vi "RIGOL DM3058 Read Single.vi"() -> ()   [LabVIEW 2018]
doc: "This example shows how to configure a measurement and take a reading."
uses:
  <instrlib>/RIGOL DM3058/RIGOL DM3058.lvlib
panel:
  in  "Auto Range (T: Enable)":bool=TRUE
  in  "Manual Range (1.0)":dbl=1.0
  in  "Function (0: DC Volts)":u16(ring) items=["DC Volts", "AC Volts", "DC Current", "AC Current", "2-Wire Resistance", "4-Wire Resistance"]
  out "Measurement":dbl
  in  "VISA resource name":refnum<visa-resource-name>
  # "(c) 2009-2015, RIGOL Technologies, Inc.  All Rights Reserved."
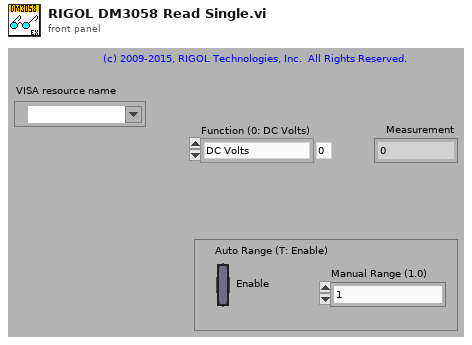
[diagram p1: front panel]
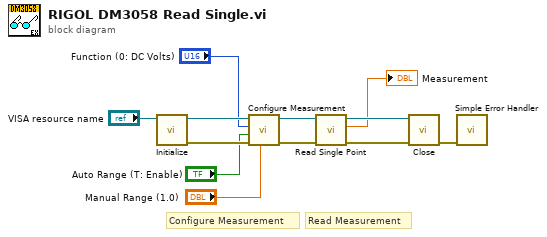
[diagram p0: block diagram]
diagram:
  # "Read Measurement"
  # "Configure Measurement"
  n1 = call <instrlib>:"Initialize.vi"("VISA resource name"="VISA resource name") -> ("error out"=w9:errorcluster, "VISA resource name out"=w10:refnum<visa-resource-name>)  [unwired: 4 in, 5 out]
  n2 = call <instrlib>:"Configure Measurement.vi"("Manual Range (1.00)"="Manual Range (1.0)", "error in (no error)"=w9, "Auto Range (T:Enable)"="Auto Range (T: Enable)", "Function (0: DC Volts)"="Function (0: DC Volts)", "VISA resource name"=w10) -> ("error out"=w4:errorcluster, "VISA resource name out"=w5:refnum<visa-resource-name>)  [unwired: 1 in, 4 out]
  n3 = call <instrlib>:"Read Single Point.vi"("error in (no error)"=w4, "VISA resource name"=w5) -> ("error out"=w2:errorcluster, "Measurement"=→"Measurement":dbl, "VISA resource name out"=w3:refnum<visa-resource-name>)  [unwired: 7 out]
  n4 = call <instrlib>:"Close.vi"("error in (no error)"=w2, "VISA resource name"=w3) -> ("error out"=w12:errorcluster)  [unwired: 9 out]
  n5 = call <vilib>:"Simple Error Handler.vi"("error in (no error)"=w12) -> ()  [unwired: 1 in, 8 out]
